vi "Get PID Settings.vi"(11 "ILC Actuator Cylinder in":refnum<class "ILC Actuator Cylinder.lvclass">) -> (2 "PID Settings":T1={"Pressure Servo Valve Settings"={"P"=1.0, "I"=0.1, "D"=0.0, "Minimum"=0.0, "Maximum"=10.0}, "Turbo Valve Settings"={"P"=1.0, "I"=0.1, "D"=0.0, "Minimum"=0.0, "Maximum"=10.0}} {"Turbo Valve Settings"."Maximum" format="%.6f"; "Turbo Valve Settings"."Minimum" format="%.6f"; "Turbo Valve Settings"."D" format="%.6f"; "Turbo Valve Settings"."I" format="%.6f"; "Turbo Valve Settings"."P" format="%.6f"; "Pressure Servo Valve Settings"."Maximum" format="%.6f"; "Pressure Servo Valve Settings"."Minimum" format="%.6f"; "Pressure Servo Valve Settings"."D" format="%.6f"; "Pressure Servo Valve Settings"."I" format="%.6f"; "Pressure Servo Valve Settings"."P" format="%.6f"}, 3 "ILC Actuator Cylinder out":refnum<class "ILC Actuator Cylinder.lvclass">)   [LabVIEW 2015, in "ILC Actuator Cylinder.lvclass"]
uses:
  ILC Actuator Cylinder.lvclass
  Typedefs/PID Settings.ctl
  Typedefs/Closed Loop Settings.ctl
  ILC Actuator Cylinder.lvclass/ILC Actuator Cylinder.ctl
  Typedefs/FAMT Typedefs.lvlib
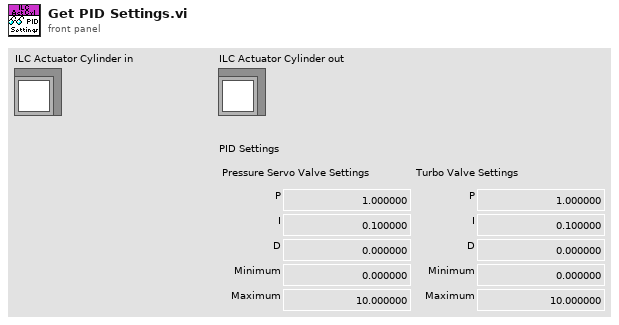
[diagram p1: front panel]
types:
  T1 = typedef "FAMT Typedefs.lvlib/PID Settings.ctl" = cluster{"Pressure Servo Valve Settings":T2, "Turbo Valve Settings":T2}
  T2 = typedef "FAMT Typedefs.lvlib/Closed Loop Settings.ctl" = cluster{"P":dbl, "I":dbl, "D":dbl, "Minimum":dbl, "Maximum":dbl}
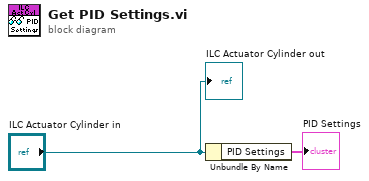
[diagram p0: block diagram]
diagram:
  n1 = Unbundle By Name("ILC Actuator Cylinder in") -> ("PID Settings"=→"PID Settings":T1)
  "ILC Actuator Cylinder out" <- "ILC Actuator Cylinder in"
